vi "UTIL Voltage to Temp.vi"(8 "Temperature Units (C)":u16(ring) items=["Celsius", "Fahrenheit", "Kelvin", "Rankine"], 11 "Voltage":waveform(dbl)={"t0"=timestamp(0 s since 1904-01-01), "dt"=0.0, "Y"=[]}) -> (3 "Temp":dbl)   [LabVIEW 2010]
uses:
  <vilib>/Analysis/NI_AALBase.lvlib
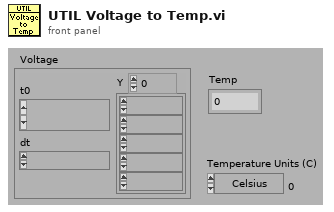
[diagram p1: front panel]
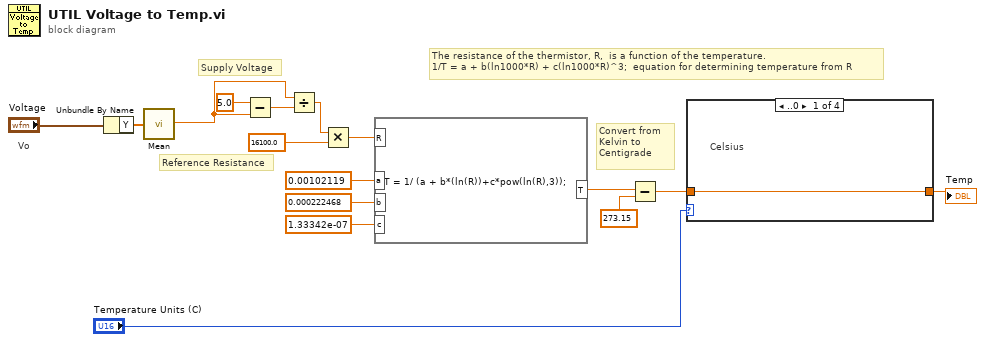
[diagram p0: block diagram]
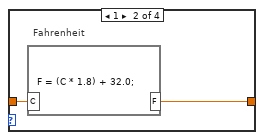
[diagram p2: hidden frame]
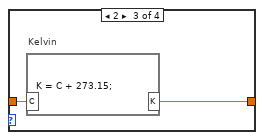
[diagram p3: hidden frame]
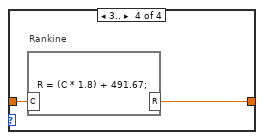
[diagram p4: hidden frame]
diagram:
  # "Convert from \nKelvin to \nCentigrade"
  # "The resistance of the thermistor, R,  is a function of the temperature.\n1/T = a + b(ln1000*R) + c(ln1000*R)^3;  equation for determining temperature from R"
  # "Reference Resistance"
  # "Supply Voltage"
  # "Vo"
  n1 = Unbundle By Name("Voltage") -> ("Y"=w4:dbl[])
  n2 = call <vilib>:"Mean.vi"("X"=w4) -> ("mean"=w2:dbl)  [unwired: 1 out]
  n3 = Subtract(x=5.0, y=w2) -> (x-y=w7:dbl)
  n4 = Divide(x=w2, y=w7) -> (x/y=w9:dbl)
  n5 = Multiply(x=w9, y=16100.0) -> (x*y=w3:dbl)
  n6 = formula code="T = 1/ (a + b*(ln(R))+c*pow(ln(R),3));"("a"=0.00102119, "b"=0.000222468, "c"=1.33342e-07, "R"=w3) -> ("T"=w12:dbl)
  n7 = Subtract(x=w12, y=273.15) -> (x-y=w10:dbl)
  n8 = case shown="..0" "Temperature Units (C)" {
    tunnel: w10 -> [w17 w19 w21 w23]
    tunnel: [w17 w18 w20 w22] -> w6
    frame ..0 {
      # "Celsius"
    }
    frame 1 {
      # "Fahrenheit"
      n9 = formula code="F = (C * 1.8) + 32.0;"("C"=w19) -> ("F"=w18:dbl)
    }
    frame 2 {
      # "Kelvin"
      n10 = formula code="K = C + 273.15;"("C"=w21) -> ("K"=w20:dbl)
    }
    frame 3.. {
      # "Rankine"
      n11 = formula code="R = (C * 1.8) + 491.67;"("C"=w23) -> ("R"=w22:dbl)
    }
  }
  "Temp" <- w6
